vi "CV.vi"() -> ()   [LabVIEW 2023]
uses:
  Sub_Vi/TypeDefsControls/Voltage.ctl
  Sub_Vi/TypeDefsControls/Iterator.ctl
  Sub_Vi/TypeDefs/WayPointCluster.ctl
  Sub_Vi/TypeDefs/ChangeOnFly.ctl
  Sub_Vi/TypeDefs/Settings.ctl
  Sub_Vi/TypeDefs/Display.ctl
  Sub_Vi/TypeDefsControls/Voltage Scan Rate.ctl
  Sub_Vi/TypeDefsControls/Time.ctl
  Settings.vi
panel:
  in  "Output Channel":u16(ring) items=["Voltage 1 (AO3)", "Voltage 2 (AO4)"]
  in  "Quiet Time (s)":T1 min=0.0
  in  "Scan Rate (V/s)":T2=0.2 min=0.0 max=1000.0
  in  "Second Voltage (V)":T3=1.0 min=-10.0 max=10.0
  in  "First Voltage (V)":T3=-1.0 min=-10.0 max=10.0
  in  "Start scan Button":bool
  in  "Jump at Start":bool
  in  "Display Cluster":T4
  in  "SettingsCluster":T5={"Sample Rate (us)"=1, "Samples Per Data Point (int, power of 2)"=1000, "DistanceToBulk (um)"=-1.0, "HoldTimeScaler"=1, "SaveData"=TRUE, "DistanceToBulk (um) 2"=-1.0, "DistanceToBulk (um) 3"=-1.0}
  in  "ChangeonFly":T6
  in  "WayPointCluster":T7
  in  "Tab Control":enum32{"V vs C1", "V vs C2", "V vs C3"}(tab)
  out "V vs C1":cluster{"Y":dbl[], "Y":dbl[]}[](graph)
  out "V vs C2":cluster{"Y":dbl[], "Y":dbl[]}[](graph)
  out "V vs C3":cluster{"Y":dbl[], "Y":dbl[]}[](graph)
  in  "Number of Cycles":T8=1.0 min=1.0
  in  "Start Voltage (V)":T3 min=-10.0 max=10.0
  in  "stop":bool
  # "Settings"
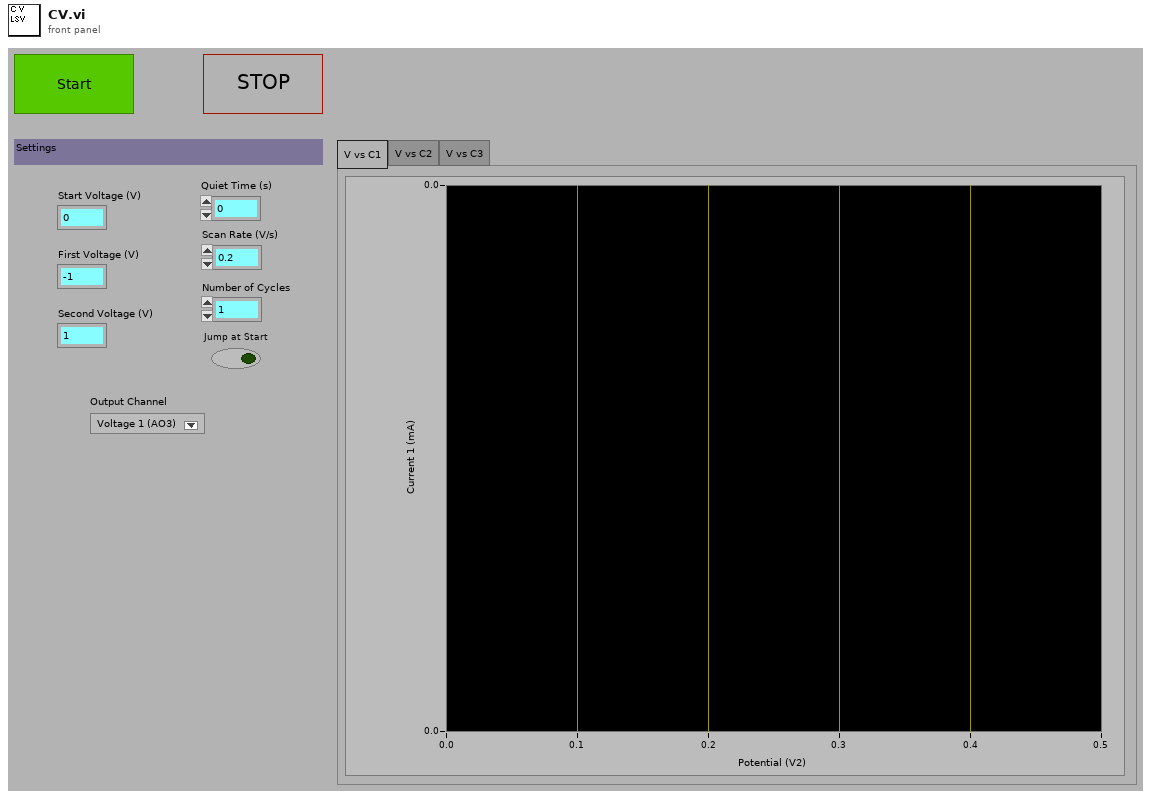
[diagram p1: front panel]
types:
  T1 = typedef "Time.ctl" = dbl
  T2 = typedef "Voltage Scan Rate.ctl" = dbl
  T3 = typedef "Voltage.ctl" = dbl
  T4 = typedef "Display.ctl" = cluster{"X":refnum<vi>, "Y":refnum<vi>, "Z":refnum<vi>, "Amp":refnum<vi>, "Phase":refnum<vi>, "t vs Z":refnum<vi>, "t vs C1":refnum<vi>, "t vs C2":refnum<vi>, "t vs C3":refnum<vi>, "t vs Amp":refnum<vi>, "t vs Phase":refnum<vi>, "t vs X":refnum<vi>, "t vs Y":refnum<vi>, "Z vs C1":refnum<vi>, "Z vs C2":refnum<vi>, "Z vs C3":refnum<vi>, "V vs C1":refnum<vi>, "V vs C2":refnum<vi>, "V vs C3":refnum<vi>, "X/Y/Z F":refnum<vi>, "X/Y/Z R":refnum<vi>, "X/Y/C1 F":refnum<vi>, "X/Y/C1 R":refnum<vi>, "X/Y/C2 F":refnum<vi>, "X/Y/C2 R":refnum<vi>, "X/Y/C3 F":refnum<vi>, "X/Y/C3 R":refnum<vi>, "NumberOfLines":u16, "um Per Pixel":dbl, "um Per Line":dbl, "X Center":dbl, "Hop X/Y/Z":refnum<vi>, "Hop X/Y/C1":refnum<vi>, "Hop X/Y/C2":refnum<vi>, "Hop X/Y/C3":refnum<vi>, "X Width":dbl, "Y Width":dbl, "Hopping Distance":dbl, "V2 vs C1":refnum<vi>, "V vs Phase":refnum<vi>, "Y Center":dbl, "Number of Pixels":dbl, "V2 vs C2":refnum<vi>, "V2 vs C3":refnum<vi>, "V vs y":refnum<vi>, "V2 vs y":refnum<vi>, "Z vs Amp":refnum<vi>, "Z vs Phase":refnum<vi>}
  T5 = typedef "Settings.ctl" = cluster{"Sample Rate (us)":u32, "Samples Per Data Point (int, power of 2)":i16, "DistanceToBulk (um)":dbl, "HoldTimeScaler":u64, "SaveData":bool, "DistanceToBulk (um) 2":dbl, "DistanceToBulk (um) 3":dbl}
  T6 = typedef "ChangeOnFly.ctl" = cluster{"Stop (boolean)":refnum<vi>, "Pause (boolean)":refnum<vi>, "EndCurrentLine (boolean)":refnum<vi>, "max movement per update step (Interger, nm)":refnum<vi>, "P (float, arb)":refnum<vi>, "Feedback set point (double, Amps)":refnum<vi>, "Voltage (double, V)":refnum<vi>, "Feedback set point 2 (double, Amps)":refnum<vi>, "Stop on Greater Than 2? (boolean)":refnum<vi>, "Stop on Greater Than? (boolean)":refnum<vi>, "Voltage 2 (double, V)":refnum<vi>, "Feedback Type (enum)":refnum<vi>, "Feedback Type 2 (enum)":refnum<vi>}
  T7 = typedef "WayPointCluster.ctl" = cluster{"X (um)":dbl[], "Y (um)":dbl[], "Z (um)":dbl[], "V (V)":dbl[], "X Velocity (um s-1)":dbl[], "Y Velocity (um s-1)":dbl[], "Z Velocity (um s-1)":dbl[], "V Velocity (V s-1)":dbl[], "FeedBack Type (enum)":u16[], "Move X (boolean)":bool[], "Move Y (boolean)":bool[], "Move Z (boolean)":bool[], "Move V (boolean)":bool[], "Jump V (boolean)":bool[], "Hold (boolean)":bool[], "Hold Time":u32[], "V2 (V)":dbl[], "Move V2":bool[], "V2 Velocity (V s-1)":dbl[], "Jump V2 (boolean)":bool[], "Update z Position delta (ms)":i16[], "Hold Feedback1":bool[], "Move Z PicoMotor":bool[], " Z PicoMotor Direction":bool[], "DIO0":bool[]}
  T8 = typedef "Iterator.ctl" = dbl
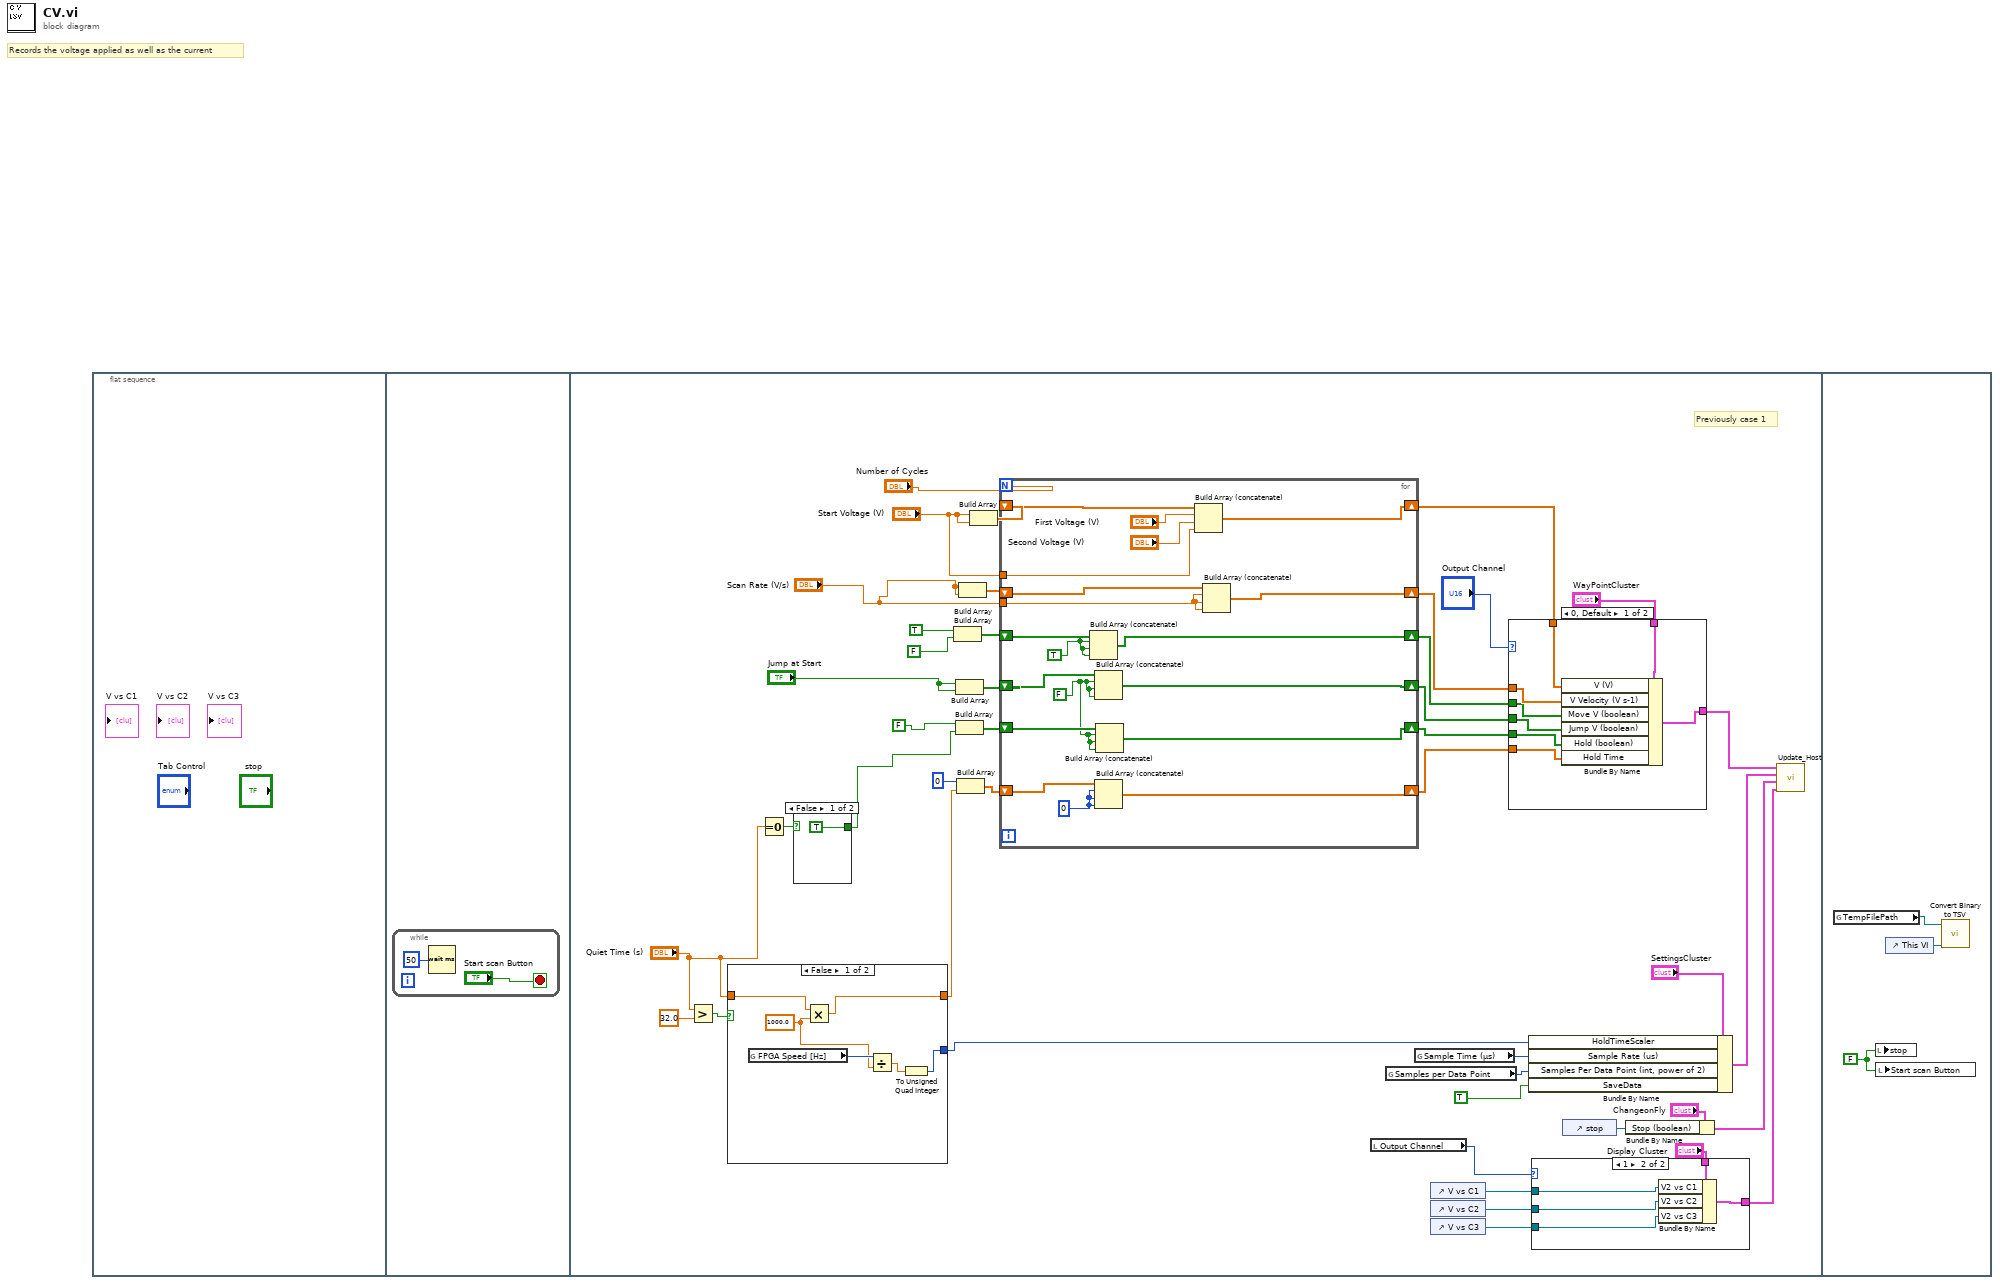
[diagram p0: block diagram]
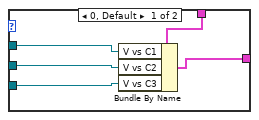
[diagram p2: hidden frame]
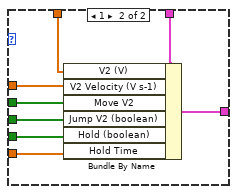
[diagram p3: hidden frame]
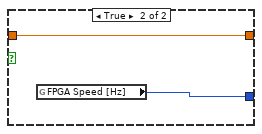
[diagram p4: hidden frame]
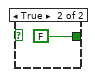
[diagram p5: hidden frame]
diagram:
  # "Records the voltage applied as well as the current"
  n1 = flat-sequence {
    frame #0 {
    }
    frame #1 {
      n2 = while {
        stop <- "Start scan Button" stop-if-true
        n3 = Wait (ms)(milliseconds to wait=u32 50) -> ()  [unwired: 1 out]
      }
    }
    frame #2 {
      # "Previously case 1"
      n4 = Greater?(x="Quiet Time (s)", y=T1 32.0) -> (0:w14:bool)
      n5 = case shown="False" w14 {
        tunnel: "Quiet Time (s)" -> [w78 w80]
        tunnel: [w77 w80] -> w12
        tunnel: [w73 w79] -> w11
        frame False {
          w75 = 1000.0 ("y")
          n6 = global read "Settings.vi" "FPGA Speed [Hz]"() -> (w76:i64)
          n7 = Multiply(x=w78, y=w75) -> (x*y=w77:T1)
          n8 = Divide(x=w76, y=w75) -> (x/y=w74:dbl)
          n9 = To Unsigned Quad Integer(1:w74) -> (0:w73:u64)
        }
        frame True {
          n10 = global read "Settings.vi" "FPGA Speed [Hz]"() -> (w79:i64)
        }
      }
      n11 = Equal To 0?(x="Quiet Time (s)") -> (x = 0?=w22:bool)
      n12 = case shown="False" w22 {
        tunnel: [TRUE ("Set Z") FALSE ("Set Z")] -> w16
        frame False {
        }
        frame True {
        }
      }
      n13 = Build Array(TRUE ("Start scan Button"), FALSE ("Start scan Button")) -> (w30:bool[])
      n14 = Build Array("Jump at Start", "Jump at Start") -> (w26:bool[])
      n15 = Build Array(FALSE ("Start scan Button"), w16) -> (w24:bool[])
      n16 = Build Array(0, w12) -> (w18:T1[])
      n17 = Build Array("Scan Rate (V/s)", "Scan Rate (V/s)") -> (w33:T2[])
      n18 = Build Array("Start Voltage (V)", "Start Voltage (V)") -> (w34:T3[])
      n19 = for {
        N: "Number of Cycles" -> [_]
        shift-right: [w100] -> w29
        shift-left: w34 -> [w101]
        shift-right: [w99] -> w28
        shift-left: w33 -> [w98]
        shift-right: [w97] -> w23
        shift-left: w26 -> [w88]
        shift-right: [w95] -> w21
        shift-left: w24 -> [w96]
        tunnel: "Start Voltage (V)" -> [w92]
        shift-right: [w90] -> w27
        shift-left: w30 -> [w91]
        shift-right: [w84] -> w17
        shift-left: w18 -> [w86]
        tunnel: "Scan Rate (V/s)" -> [w83]
        w85 = 0
        w87 = FALSE ("Start scan Button")
        w89 = TRUE ("Start scan Button")
        n20 = Build Array (concatenate)(w91, w89, w89, w89) -> (w90:bool[])
        n21 = Build Array (concatenate)(w88, w87, w87, w87) -> (w97:bool[])
        n22 = Build Array (concatenate)(w86, w85, w85, w85) -> (w84:T1[])
        n23 = Build Array (concatenate)(w96, w87, w87, w87) -> (w95:bool[])
        n24 = Build Array (concatenate)(w101, "First Voltage (V)", "Second Voltage (V)", w92) -> (w100:T3[])
        n25 = Build Array (concatenate)(w98, w83, w83, w83) -> (w99:T2[])
      }
      n26 = local read "Output Channel"() -> (w5:u16)
      n27 = global read "Settings.vi" "Samples per Data Point"() -> (w36:u16)
      n28 = global read "Settings.vi" "Sample Time (µs)"() -> (w41:u32)
      n29 = control-ref of="V vs C1"() -> (w6:refnum<vi>)
      n30 = control-ref of="V vs C2"() -> (w4:refnum<vi>)
      n31 = control-ref of="V vs C3"() -> (w3:refnum<vi>)
      n32 = case shown="0, Default" "Output Channel" {
        tunnel: "WayPointCluster" -> [w57 w72]
        tunnel: [w58 w71] -> w40
        tunnel: w29 -> [w64 w70]
        tunnel: w28 -> [w63 w69]
        tunnel: w27 -> [w62 w68]
        tunnel: w23 -> [w61 w67]
        tunnel: w21 -> [w60 w66]
        tunnel: w17 -> [w59 w65]
        frame 0, Default {
          n33 = Bundle By Name(cluster=w57, "V (V)"=w64, "V Velocity (V s-1)"=w63, "Move V (boolean)"=w62, "Jump V (boolean)"=w61, "Hold (boolean)"=w60, "Hold Time"=w59) -> (w58:T7)
        }
        frame 1 {
          n34 = Bundle By Name(cluster=w72, "V2 (V)"=w70, "V2 Velocity (V s-1)"=w69, "Move V2"=w68, "Jump V2 (boolean)"=w67, "Hold (boolean)"=w66, "Hold Time"=w65) -> (w71:T7)
        }
      }
      n35 = Bundle By Name(cluster="SettingsCluster", "HoldTimeScaler"=w11, "Sample Rate (us)"=w41, "Samples Per Data Point (int, power of 2)"=w36, "SaveData"=TRUE) -> (w38:T5)
      n36 = case shown="1" w5 {
        tunnel: "Display Cluster" -> [w51 w56]
        tunnel: [w50 w55] -> w39
        tunnel: w6 -> [w49 w54]
        tunnel: w4 -> [w48 w53]
        tunnel: w3 -> [w47 w52]
        frame 0, Default {
          n37 = Bundle By Name(cluster=w51, "V vs C1"=w49, "V vs C2"=w48, "V vs C3"=w47) -> (w50:T4)
        }
        frame 1 {
          n38 = Bundle By Name(cluster=w56, "V2 vs C1"=w54, "V2 vs C2"=w53, "V2 vs C3"=w52) -> (w55:T4)
        }
      }
      n39 = control-ref of="stop"() -> (w46:refnum<vi>)
      n40 = Bundle By Name(cluster="ChangeonFly", "Stop (boolean)"=w46) -> (w37:T6)
      n41 = call "Update_Host.vi"("Display Cluster"=w39, "ChangeonFly"=w37, "SettingsCluster"=w38, "WayPointCluster"=w40) -> ()  [unwired: 6 in]
    }
    frame #3 {
      w104 = FALSE ("Start scan Button")
      n42 = global read "Settings.vi" "TempFilePath"() -> (w102:path)
      n43 = local write "stop"(w104) -> ()
      n44 = local write "Start scan Button"(w104) -> ()
      n45 = control-ref of="This VI"() -> (w103:refnum<vi>)
      n46 = call "Convert Binary to TSV.vi"("This VI"=w103, "TDMS DataFile Name"=w102) -> ()  [unwired: 10 in]
    }
  }
